vi "Register.vi"() -> ()   [LabVIEW 2024, in "GUI.lvlib"]
uses:
  <vilib>/addons/_JKI.lib/REST Client/classes/REST Client/HTTP Header.ctl
  <vilib>/NI/Advanced HTTP Client/Header--Combo Box.ctl
  <vilib>/addons/_JKI.lib/REST Client/classes/REST Client/REST Client.lvclass
  GUI.lvlib
  <vilib>/NI/Advanced HTTP Client/Session.lvclass
  <userlib>/FTools/JSON Pretty Printer/JSON Pretty Printer.lvlib
panel:
  in  "Faction":string
  in  "user":string
  out "error out 2":errorcluster
  out "Status String":string
  out "Response body":string
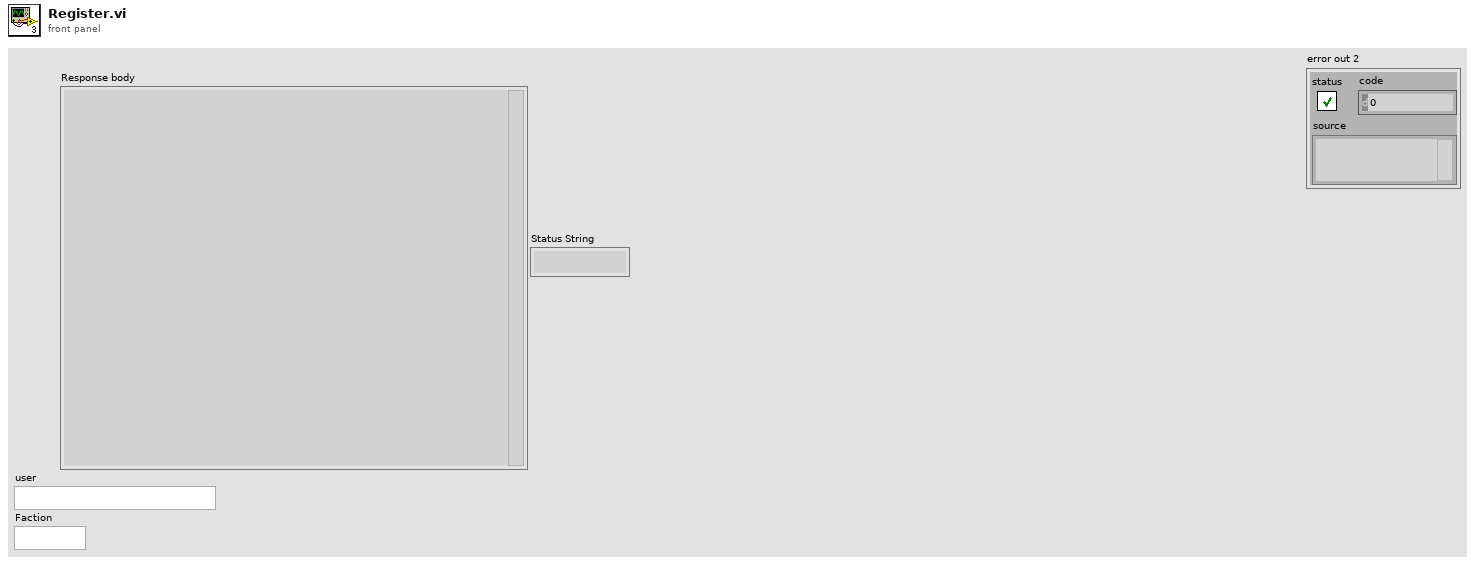
[diagram p1: front panel]
types:
  T1 = typedef "lib_NI_Advanced HTTP Client.lvlib/Session.lvclass/Header--Combo Box.ctl" = string
  T2 = typedef "REST Client.lvlib/REST Client.lvclass/HTTP Header.ctl" = cluster{"header":T1, "value":string}
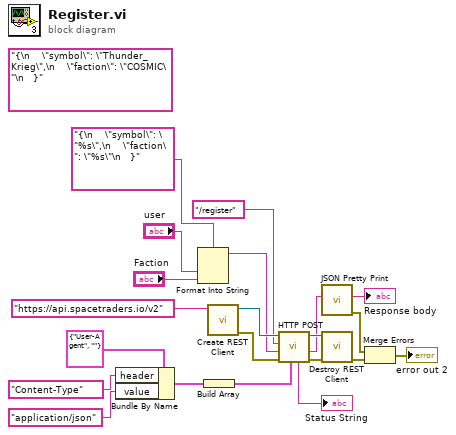
[diagram p0: block diagram]
diagram:
  (unwired) "{\n    \"symbol\": \"Thunder_Krieg\",\n    \"faction\": \"COSMIC\"\n   }" ("Request body")
  n1 = Bundle By Name(cluster=T2 {"header"="User-Agent", "value"=""} ("Header"), "header"=T1 "Content-Type", "value"="application/json") -> (w18:T2)
  n2 = Format Into String(format string="{\n    \"symbol\": \"%s\",\n    \"faction\": \"%s\"\n   }" ("Request body"), "user", "Faction") -> (resulting string=w8:string)  [unwired: 2 in, 1 out]
  n3 = Build Array(w18) -> (w17:T2[])
  n4 = call <vilib>:"Create REST Client.vi"("Base URL"="https://api.spacetraders.io/v2") -> ("error out"=w13:errorcluster, "REST Client out"=w15:refnum<class "REST Client.lvclass">)  [unwired: 9 in]
  n5 = call-dynamic "HTTP POST.vi"("request specific headers"=w17, "error in (no error)"=w13, "Request body"=w8, "Path"="/register", "REST Client in"=w15) -> ("error out"=w11:errorcluster, "Response body"=w4:string, "REST Client out"=w14:refnum<class "REST Client.lvclass">, "Status String"=→"Status String":string)  [unwired: 1 in, 2 out]
  n6 = call <userlib>:"JSON Pretty Print.vi"("JSON String"=w4) -> ("error out"=w1:errorcluster, "JSON Pretty Print Format"=→"Response body":string)  [unwired: 9 in]
  n7 = call-dynamic "Destroy REST Client.vi"("error in (no error)"=w11, "REST Client in"=w14) -> ("error out"=w20:errorcluster)  [unwired: 9 in]
  n8 = Merge Errors(w1, w20) -> (→"error out 2":errorcluster)
